vi "230524_ExamPractice.vi"() -> ()   [LabVIEW 2022 SP3]
uses:
  <vilib>/addons/database/Connection.llb/DB Tools Open Connec (Path).vi
  <vilib>/addons/database/_DB Variant To Data/Database Variant To Data.xnode
  <vilib>/addons/database/NI_Database_API.lvlib
panel:
  in  "Enum":enum16{"lieferant", "art_einzel", "art_ges"}(ring)
  in  "stop":bool
  in  "connection information":path=path "D:/School/AIIT/4AHME/LabView/230524_ExamPractice/230524_ExamPractice.udl"
  in  "Tab Control":enum32{"Lesen", "Schreiben"}(tab)
  out "data":string[][](array[string])
  in  "Write":bool
  in  "lnr":string
  in  "firmenname":string
  in  "plz":string
  in  "ort":string
  in  "strasse":string
  in  "strasse_nr":string
  in  "vertreter":string
  in  "vertreter_tel_nr":string
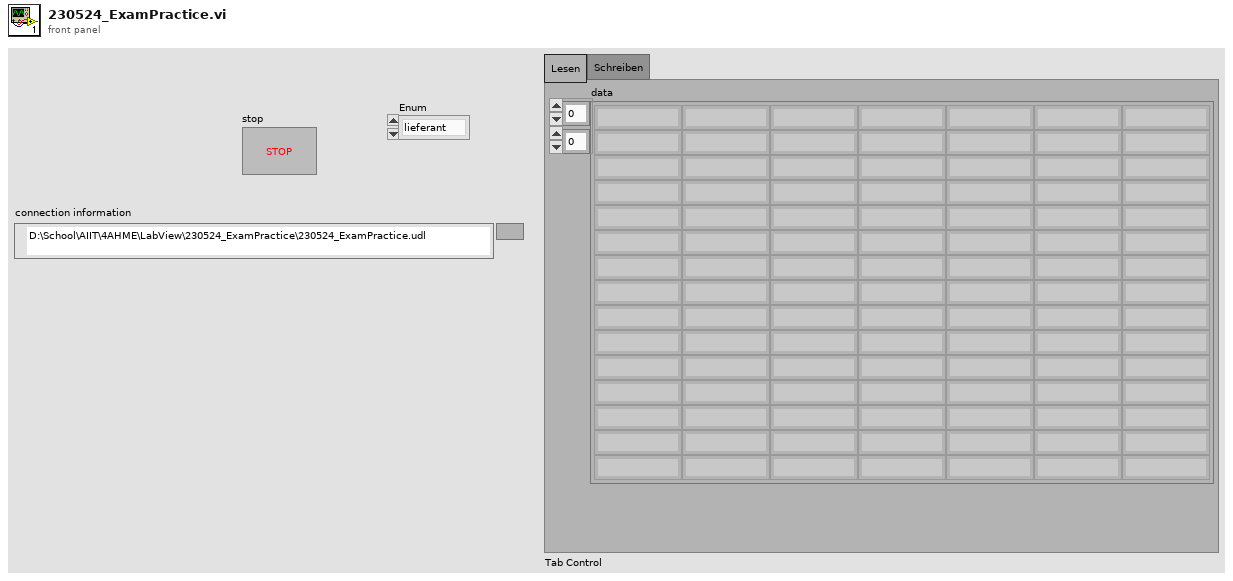
[diagram p1: front panel]
types:
  T1 = cluster{"lnr":string, "firmenname":string, "plz":string, "ort":string, "strasse":string, "strasse_nr":string, "vertreter":string, "vertreter_tel_nr":string}
  T2 = typedef "NI_Database_API.lvlib/Conn ObjectReference.ctl" = refnum<k1>
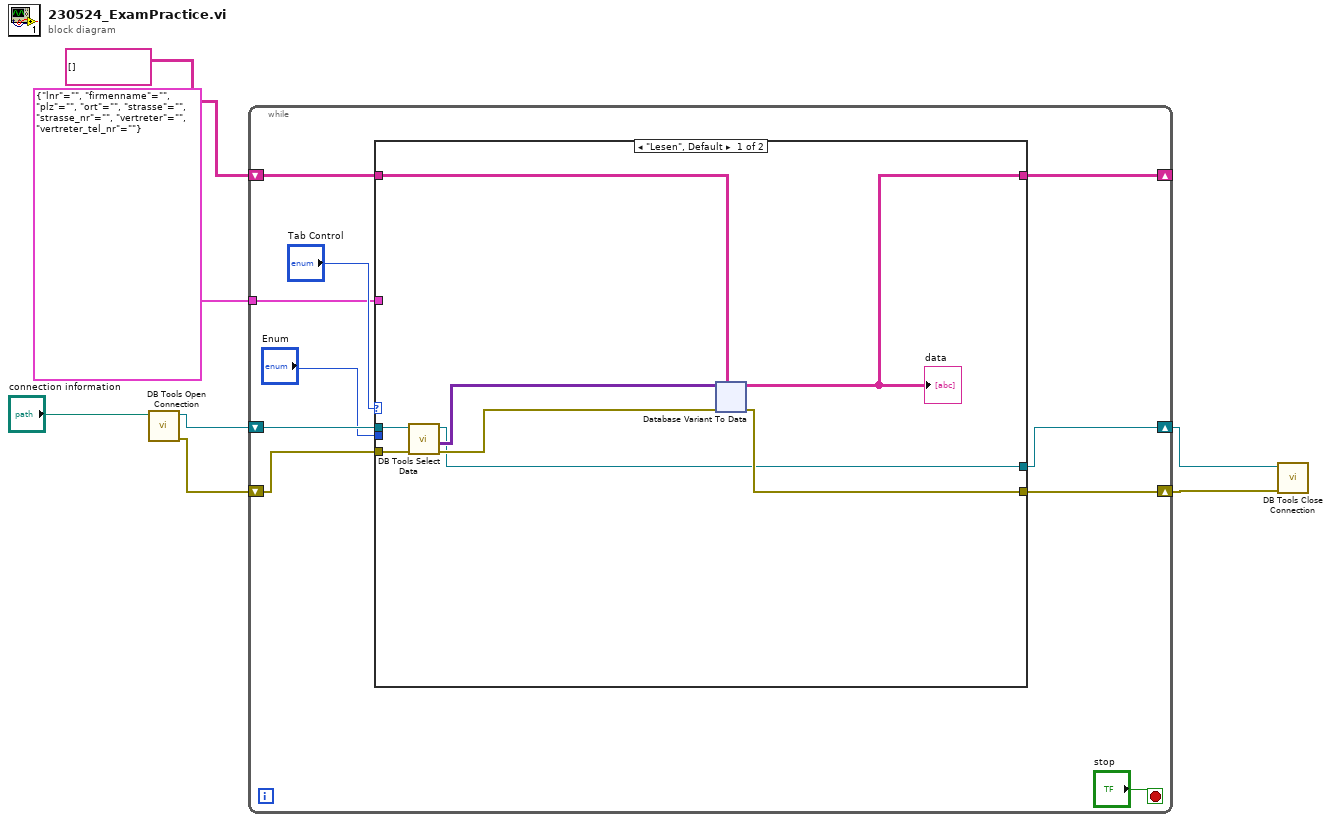
[diagram p0: block diagram]
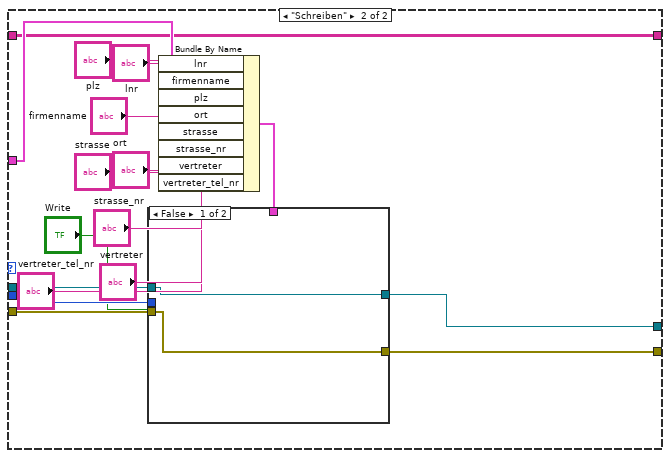
[diagram p2: hidden frame]
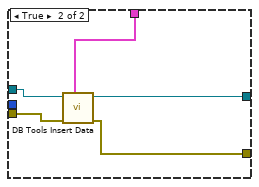
[diagram p3: hidden frame]
diagram:
  n1 = call-poly <vilib>:"DB Tools Open Connection.vi"("connection information"="connection information") -> ("error out"=w5:errorcluster, "connection reference"=w6:T2)  [unwired: 7 in]
  n2 = while {
    shift-right: [w15] -> w4
    shift-left: w5 -> [w16]
    shift-right: [w10] -> w1
    shift-left: w6 -> [w17]
    tunnel: T1 {"lnr"="", "firmenname"="", "plz"="", "ort"="", "strasse"="", "strasse_nr"="", "vertreter"="", "vertreter_tel_nr"=""} -> [w11]
    shift-right: [w9] -> _
    shift-left: string[][] [] -> [w13]
    stop <- "stop" stop-if-true
    n3 = case shown="\"Lesen\", Default" "Tab Control" {
      tunnel: w17 -> [w25 w81]
      tunnel: w16 -> [w24 w83]
      tunnel: [w22 w86] -> w15
      tunnel: "Enum" -> [_ w84]
      tunnel: w13 -> [w20 w78]
      tunnel: [w19 w85] -> w10
      tunnel: w11 -> [_ w80]
      tunnel: [w18 w78] -> w9
      frame "Lesen", Default {
        n4 = call <vilib>:"DB Tools Select Data.vi"("error in (no error)"=w24, "connection reference"=w25) -> ("error out"=w23:errorcluster, "data"=w21:variant[][], "connection reference out"=w19:T2)  [unwired: 4 in]
        n5 = xnode "Database Variant To Data"("database variant"=w21, "error in (no error)"=w23, "type"=w20) -> ("data"=w18:string[][], "error out"=w22:errorcluster)
        "data" <- w18
      }
      frame "Schreiben" {
        n6 = Bundle By Name(cluster=w80, "lnr"="lnr", "firmenname"="firmenname", "plz"="plz", "ort"="ort", "strasse"="strasse", "strasse_nr"="strasse_nr", "vertreter"="vertreter", "vertreter_tel_nr"="vertreter_tel_nr") -> (w79:T1)
        n7 = case shown="False" "Write" {
          tunnel: [w88 w93] -> w86
          tunnel: [w87 w92] -> w85
          tunnel: w84 -> [_ _]
          tunnel: w83 -> [w88 w91]
          tunnel: w81 -> [w87 w90]
          tunnel: w79 -> [_ w89]
          frame False {
          }
          frame True {
            n8 = call <vilib>:"DB Tools Insert Data.vi"("data"=w89, "error in (no error)"=w91, "connection reference"=w90) -> ("error out"=w93:errorcluster, "connection reference out"=w92:T2)  [unwired: 7 in]
          }
        }
      }
    }
  }
  n9 = call <vilib>:"DB Tools Close Connection.vi"("error in (no error)"=w4, "connection reference"=w1) -> ()  [unwired: 5 in, 1 out]
